vi "File_Merger.vi"() -> ()   [LabVIEW 2019]
uses:
  <vilib>/Utility/file.llb/Read Delimited Spreadsheet (string).vi
  <vilib>/Utility/file.llb/Write Delimited Spreadsheet (string).vi
panel:
  out "Total_Files":i32
  out "Processing_File":i32
  out "CSV_Files":path[](array[path])
  out "type":string
  out "All Files in Dir":path[](array[path])
  out "Output_File":path
  in  "Folder":path
  in  "error in (no error)":errorcluster
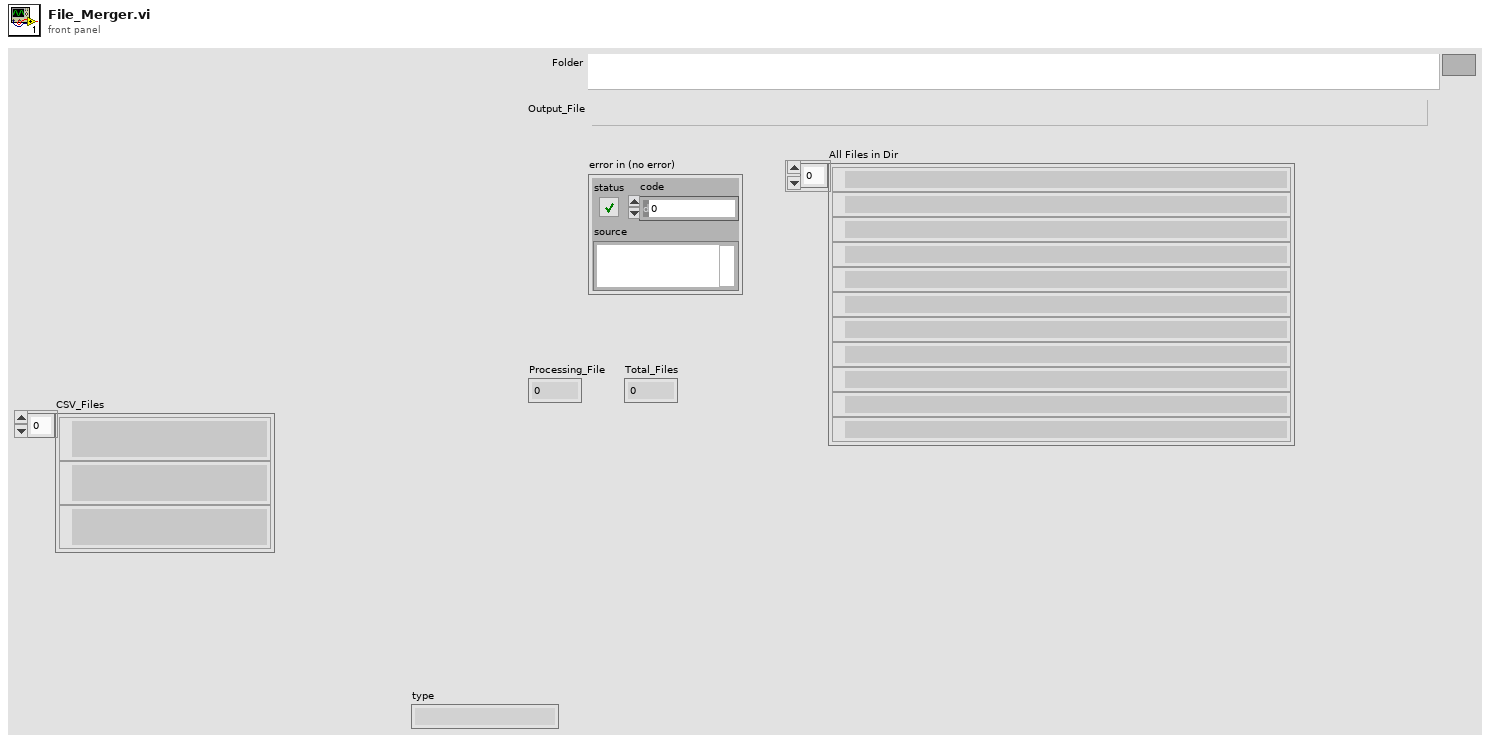
[diagram p1: front panel]
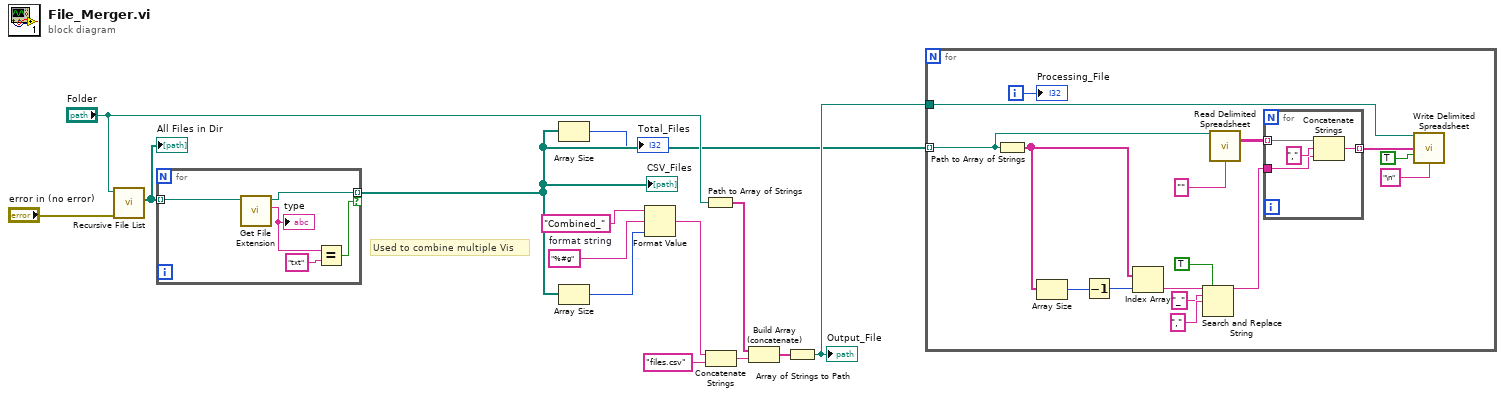
[diagram p0: block diagram]
diagram:
  w4 = "%#g"  # format string
  # "Used to combine multiple Vis"
  n1 = call <vilib>:"Recursive File List.vi"("error in (no error)"="error in (no error)", "Folder Path"="Folder") -> ("All Files in Dir"=w14:path[])  [unwired: 5 in, 4 out]
  "All Files in Dir" <- w14
  n2 = for {
    tunnel: w14 -> [w17] mode=indexing
    tunnel: [w16] -> w2 mode=indexing if=w15
    n3 = call <vilib>:"Get File Extension.vi"("file"=w17) -> ("lowercase file extension"=w19:string, "dup file"=w16:path)  [unwired: 6 in, 3 out]
    "type" <- w19
    n4 = Equal?(x=w19, y="txt") -> (x = y?=w15:bool)
  }
  "CSV_Files" <- w2
  n5 = Array Size(array=w2) -> (size(s)=→"Total_Files":i32)
  n6 = Array Size(array=w2) -> (size(s)=w11:i32)
  n7 = Format Value(string ("")="Combined_" ("y"), format string=w4, value (0)=w11) -> (output string=w6:string)
  n8 = Path to Array of Strings(0:"Folder") -> (2:w10:string[])  [unwired: 1 out]
  n9 = Concatenate Strings(w6, "files.csv" ("y")) -> (w7:string)
  n10 = Build Array (concatenate)(w10, w7) -> (w9:string[])
  n11 = Array of Strings to Path(0:w9) -> (2:w8:path)  [unwired: 1 in]
  "Output_File" <- w8
  n12 = for {
    tunnel: w2 -> [w27] mode=indexing
    tunnel: w8 -> [w21]
    i -> [w20]
    n13 = Path to Array of Strings(0:w27) -> (2:w24:string[])  [unwired: 1 out]
    n14 = Array Size(array=w24) -> (size(s)=w26:i32)
    n15 = Decrement(x=w26) -> (x-1=w25:i32)
    n16 = Index Array(array=w24, index=w25) -> (element=w23:string)
    n17 = Search and Replace String(replace all?=TRUE ("replace all? (F)"), input string=w23, search string="_", replace string="," ("replace string (\"\")")) -> (result string=w30:string)  [unwired: 4 in, 3 out]
    n18 = call-poly <vilib>:"Read Delimited Spreadsheet.vi"("file path (dialog if empty)"=w27, "delimiter (\\t)"="" ("delimiter (\\t)")) -> ("all rows"=w35:string[][])  [unwired: 8 in, 5 out]
    n19 = for {
      tunnel: w35 -> [w39] mode=indexing
      tunnel: w30 -> [w37]
      tunnel: [w36] -> w32 mode=indexing
      n20 = Concatenate Strings(w39, "," ("delimiter (\\t)"), w37) -> (w36:string)
    }
    n21 = call-poly <vilib>:"Write Delimited Spreadsheet.vi"("file path (dialog if empty)"=w21, "1D data"=w32, "append to file? (new file:F)"=TRUE, "delimiter (\\t)"="\n" ("delimiter (\\t)")) -> ()  [unwired: 10 in, 2 out]
    "Processing_File" <- w20
  }
